vi "Assert To Report Entry.vi"(8 "error in (no error)":errorcluster, 10 "Assert":T1={"Name"="", "Passed"=FALSE, "Call Chain"=[], "Test Error"={"status"=FALSE, "code"=0, "source"=""}, "Time Stamp"=timestamp(0 s since 1904-01-01), "Unique Assert ID"="", "Test Key"="", "Execution time (s)"=-1.0, "Verbose Explanation"=""}) -> (0 "error out":errorcluster, 2 "String":string)   [LabVIEW 2013, in "Caraya.lvlib" / "Test Report.Default.lvclass"]
uses:
  Test Report.Default.lvclass
  Test Result/Assert Event Data.ctl
  Test Report/Test Report.lvclass
  Test Result/Test Result.lvclass
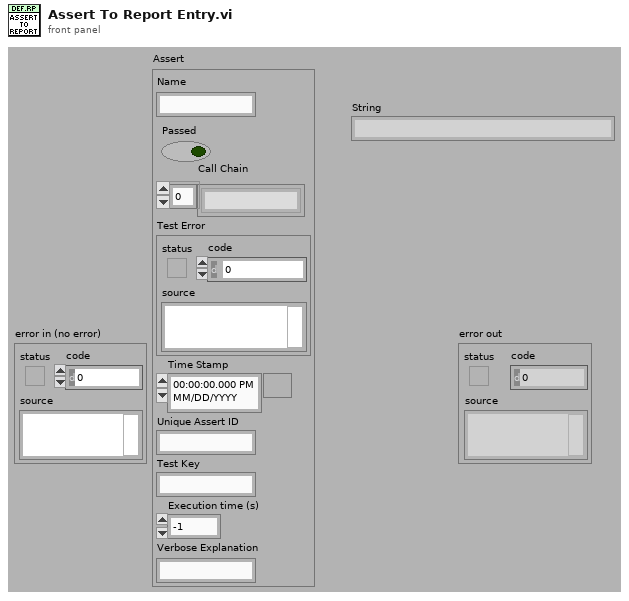
[diagram p1: front panel]
types:
  T1 = typedef "Caraya.lvlib/Test Result.lvclass/Assert Event Data.ctl" = cluster{"Name":string, "Passed":bool, "Call Chain":string[], "Test Error":errorcluster, "Time Stamp":timestamp, "Unique Assert ID":string, "Test Key":string, "Execution time (s)":dbl, "Verbose Explanation":string}
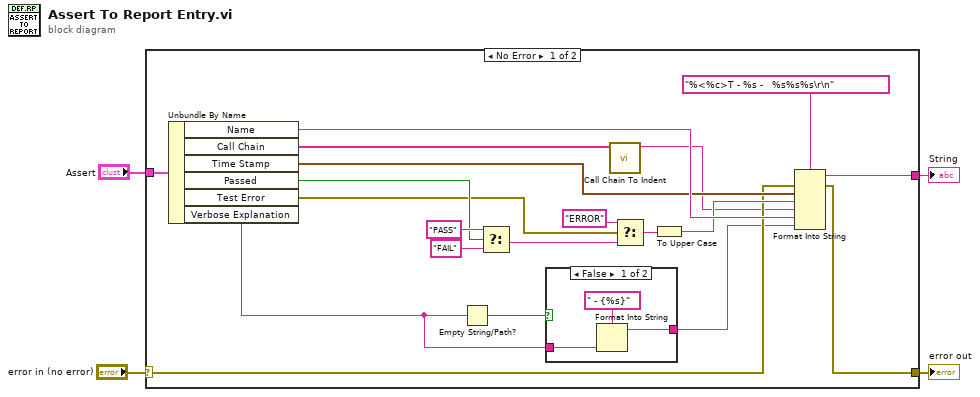
[diagram p0: block diagram]
diagram:
  n1 = case shown="No Error" "error in (no error)" {
    selector: "error in (no error)" -> [w13 w28]
    tunnel: [w22 w28] -> w3
    tunnel: "Assert" -> [w20 _]
    tunnel: [w21 _] -> w1
    frame No Error {
      n2 = Unbundle By Name(w20) -> ("Name"=w23:string, "Call Chain"=w19:string[], "Time Stamp"=w18:timestamp, "Passed"=w10:bool, "Test Error"=w9:errorcluster, "Verbose Explanation"=w7:string)
      n3 = Empty String/Path?(string/path=w7) -> (empty?=w6:bool)
      n4 = Select(t="PASS" ("format string"), s=w10, f="FAIL" ("format string")) -> (s? t:f=w12:string)
      n5 = case shown="False" w6 {
        tunnel: w7 -> [w26 _]
        tunnel: [w25 _] -> w5
        frame False {
          n6 = Format Into String(format string=" - {%s}", w26) -> (resulting string=w25:string)  [unwired: 2 in, 1 out]
        }
        frame True {
        }
      }
      n7 = call "Call Chain To Indent.vi"("Call Chain"=w19) -> ("Indent"=w8:string)  [unwired: 10 in]
      n8 = Select(t="ERROR" ("format string"), s=w9, f=w12) -> (s? t:f=w15:string)
      n9 = To Upper Case(1:w15) -> (0:w14:string)
      n10 = Format Into String(format string="%<%c>T - %s -   %s%s%s\r\n", error in=w13, w18, w14, w8, w23, w5) -> (resulting string=w21:string, error out=w22:errorcluster)  [unwired: 1 in]
    }
    frame Error {
    }
  }
  "error out" <- w3
  "String" <- w1
